vi "Update Data.vi"(8 "error in (no error)":errorcluster, 10 "Debug Data":refnum<class "Debug Data.lvclass">[](array[class]), 11 "List Seen Processes View Model In":refnum<class "List Messages View Model.lvclass">) -> (0 "error out":errorcluster, 3 "List Seen Processes View Model Out":refnum<class "List Messages View Model.lvclass">)   [LabVIEW 2020, in "List Messages View Model.lvclass"]
uses:
  List Messages View Model.lvclass
  List Messages View Model.lvclass/List Messages View Model.ctl
  Debug Data/Debug Data.lvclass
  List Box View Model_/List Box View Model.lvclass
  C:/Users/anton/Documents/GitHub/triarc-debugger/source/List Box View Model_/List Box View Model.lvclass
  C:/Users/anton/Documents/GitHub/triarc-debugger/source/List Seen Messages View Model/List Messages View Model.lvclass
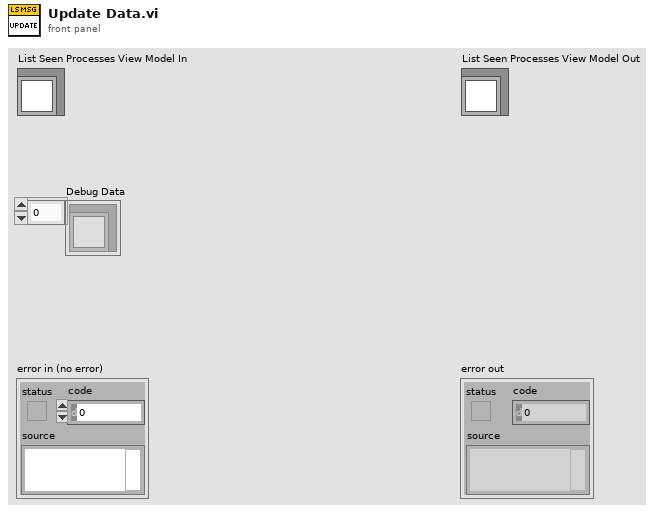
[diagram p1: front panel]
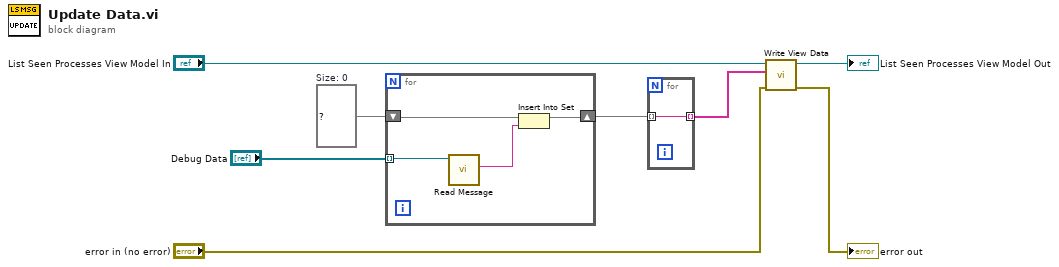
[diagram p0: block diagram]
diagram:
  w6 = set{string} {}  # Size: 0
  n1 = for {
    tunnel: "Debug Data" -> [w12] mode=indexing
    shift-right: [w9] -> w5
    shift-left: w6 -> [w11]
    n2 = call "Read Message.vi"("Debug Data in"=w12) -> ("Message"=w10:string)  [unwired: 7 in, 3 out]
    n3 = Insert Into Set(10:w10, 11:w11) -> (3:w9:set{string})  [unwired: 1 out]
  }
  n4 = for {
    tunnel: [w13] -> w1 mode=indexing
    tunnel: w5 -> [w13] mode=indexing
  }
  n5 = call "Write View Data.vi"("error in (no error)"="error in (no error)", "View Data"=w1, "List Box View Model in"="List Seen Processes View Model In") -> ("error out"=→"error out":errorcluster, "List Box View Model out"=→"List Seen Processes View Model Out":refnum<class "List Messages View Model.lvclass">)  [unwired: 7 in]
